vi "importUserPeaks.vi"(0 "iPeak_Location":dbl[](array[numeric]), 5 "amplitudePeaks":dbl[](array[numeric]), 7 "iPeak_LocationUSER":dbl[](array[numeric]), 9 "amplitudePeaksUSER":dbl[](array[numeric]), 11 "Error In":errorcluster) -> (6 "iPeak_LocationFinal":dbl[](array[numeric]), 10 "amplitudePeaksFinal":dbl[](array[numeric]), 15 "Error Out":errorcluster)   [LabVIEW 2015]
doc: "Insert in to the peaks array, that were detected by the algorithm, the peaks selected by the user."
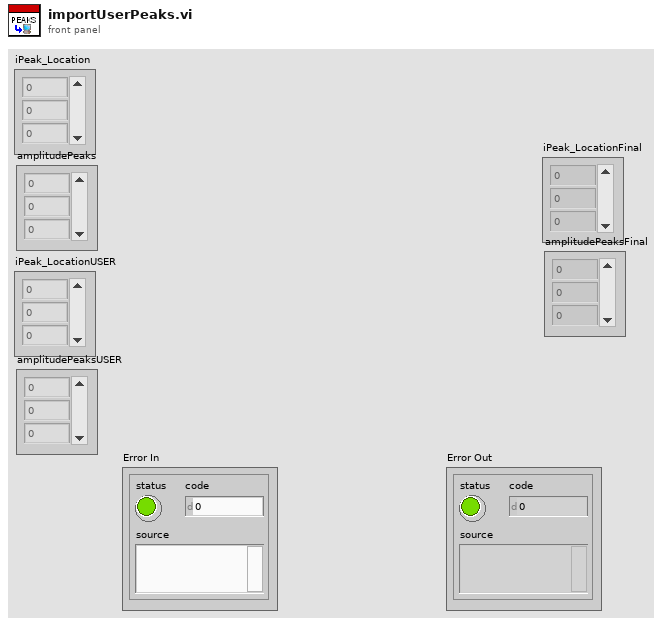
[diagram p1: front panel]
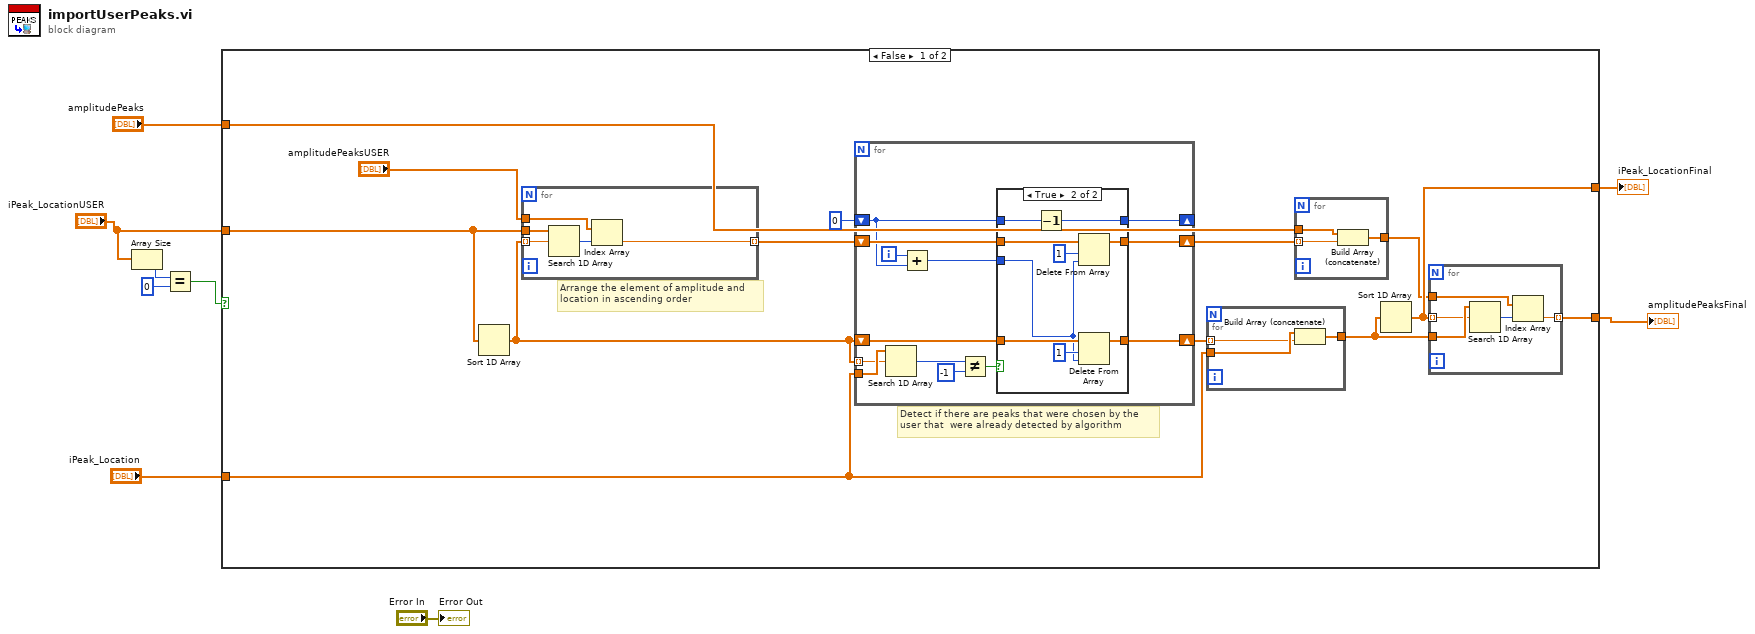
[diagram p0: block diagram]
diagram:
  n1 = Array Size(array="iPeak_LocationUSER") -> (size(s)=w3:i32)
  n2 = Equal?(x=w3, y=0) -> (x = y?=w1:bool)
  n3 = case shown="False" w1 {
    tunnel: "iPeak_Location" -> [w18 w64]
    tunnel: "amplitudePeaks" -> [w15 w65]
    tunnel: [w14 w64] -> w6
    tunnel: [w11 w65] -> w5
    tunnel: "iPeak_LocationUSER" -> [w10 _]
    frame False {
      # "Detect if there are peaks that were chosen by the \nuser that  were already detected by algorithm"
      # "Arrange the element of amplitude and\nlocation in ascending order"
      n4 = Sort 1D Array(array=w10) -> (sorted array=w19:dbl[])
      n5 = for {
        tunnel: w19 -> [w62] mode=indexing
        tunnel: w10 -> [w63]
        tunnel: "amplitudePeaksUSER" -> [w61]
        tunnel: [w59] -> w21 mode=indexing
        n6 = Search 1D Array(1D array=w63, element=w62) -> (index of element=w60:i32)  [unwired: 1 in]
        n7 = Index Array(array=w61, index=w60) -> (element=w59:dbl)
      }
      n8 = for {
        tunnel: w19 -> [w45] mode=indexing
        tunnel: w18 -> [w46]
        shift-right: [w40] -> w16
        shift-left: w21 -> [w44]
        shift-right: [w39] -> _
        shift-left: 0 -> [w36]
        shift-right: [w35] -> w17
        shift-left: w19 -> [w34]
        i -> [w37]
        n9 = Search 1D Array(1D array=w46, element=w45) -> (index of element=w43:i32)  [unwired: 1 in]
        n10 = Add(x=w37, y=w36) -> (x+y=w38:i32)
        n11 = Not Equal?(x=w43, y=-1) -> (x != y?=w41:bool)
        n12 = case shown="True" w41 {
          tunnel: w44 -> [w49 w58]
          tunnel: w38 -> [_ w50]
          tunnel: [w49 w56] -> w40
          tunnel: [w48 w55] -> w39
          tunnel: w36 -> [w48 w54]
          tunnel: [w47 w52] -> w35
          tunnel: w34 -> [w47 w51]
          frame False {
          }
          frame True {
            n13 = Decrement(x=w54) -> (x-1=w55:i32)
            n14 = Delete From Array(array=w58, length=1, index=w50) -> (array with subset deleted=w56:dbl[])  [unwired: 1 out]
            n15 = Delete From Array(array=w51, length=1, index=w50) -> (array with subset deleted=w52:dbl[])  [unwired: 1 out]
          }
        }
      }
      n16 = for {
        tunnel: w18 -> [w33]
        tunnel: w17 -> [w32] mode=indexing
        tunnel: [w31] -> w13
        n17 = Build Array (concatenate)(w33, w32) -> (w31:dbl[])
      }
      n18 = for {
        tunnel: w15 -> [w30]
        tunnel: w16 -> [w29] mode=indexing
        tunnel: [w28] -> w12
        n19 = Build Array (concatenate)(w30, w29) -> (w28:dbl[])
      }
      n20 = Sort 1D Array(array=w13) -> (sorted array=w14:dbl[])
      n21 = for {
        tunnel: w14 -> [w26] mode=indexing
        tunnel: w13 -> [w27]
        tunnel: w12 -> [w25]
        tunnel: [w23] -> w11 mode=indexing
        n22 = Search 1D Array(1D array=w27, element=w26) -> (index of element=w24:i32)  [unwired: 1 in]
        n23 = Index Array(array=w25, index=w24) -> (element=w23:dbl)
      }
    }
    frame True {
    }
  }
  "iPeak_LocationFinal" <- w6
  "amplitudePeaksFinal" <- w5
  "Error Out" <- "Error In"
